vi "GetEvents_Motor Controller.vi"(8 "error in (no error)":errorcluster, 11 "TopLevel in":refnum<class "Motor Controller.lvclass">) -> (0 "error out":errorcluster, 2 "UserEvents":T1, 3 "TopLevel out":refnum<class "Motor Controller.lvclass">)   [LabVIEW 2022 SP3, in "Motor Controller.lvclass"]
uses:
  Motor Controller.lvclass
  Typedefs/UserEvents.ctl
  Typedefs/API Event Data.ctl
  Typedefs/API Task State.ctl
  Typedefs/Status.ctl
  TopLevel/Typedefs/Motor Controller Config Data.ctl
  Typedefs/Stage Move Data.ctl
  Typedefs/Batch Index Speed Data.ctl
  Typedefs/Move Status.ctl
  Motor Controller.lvclass/Motor Controller.ctl
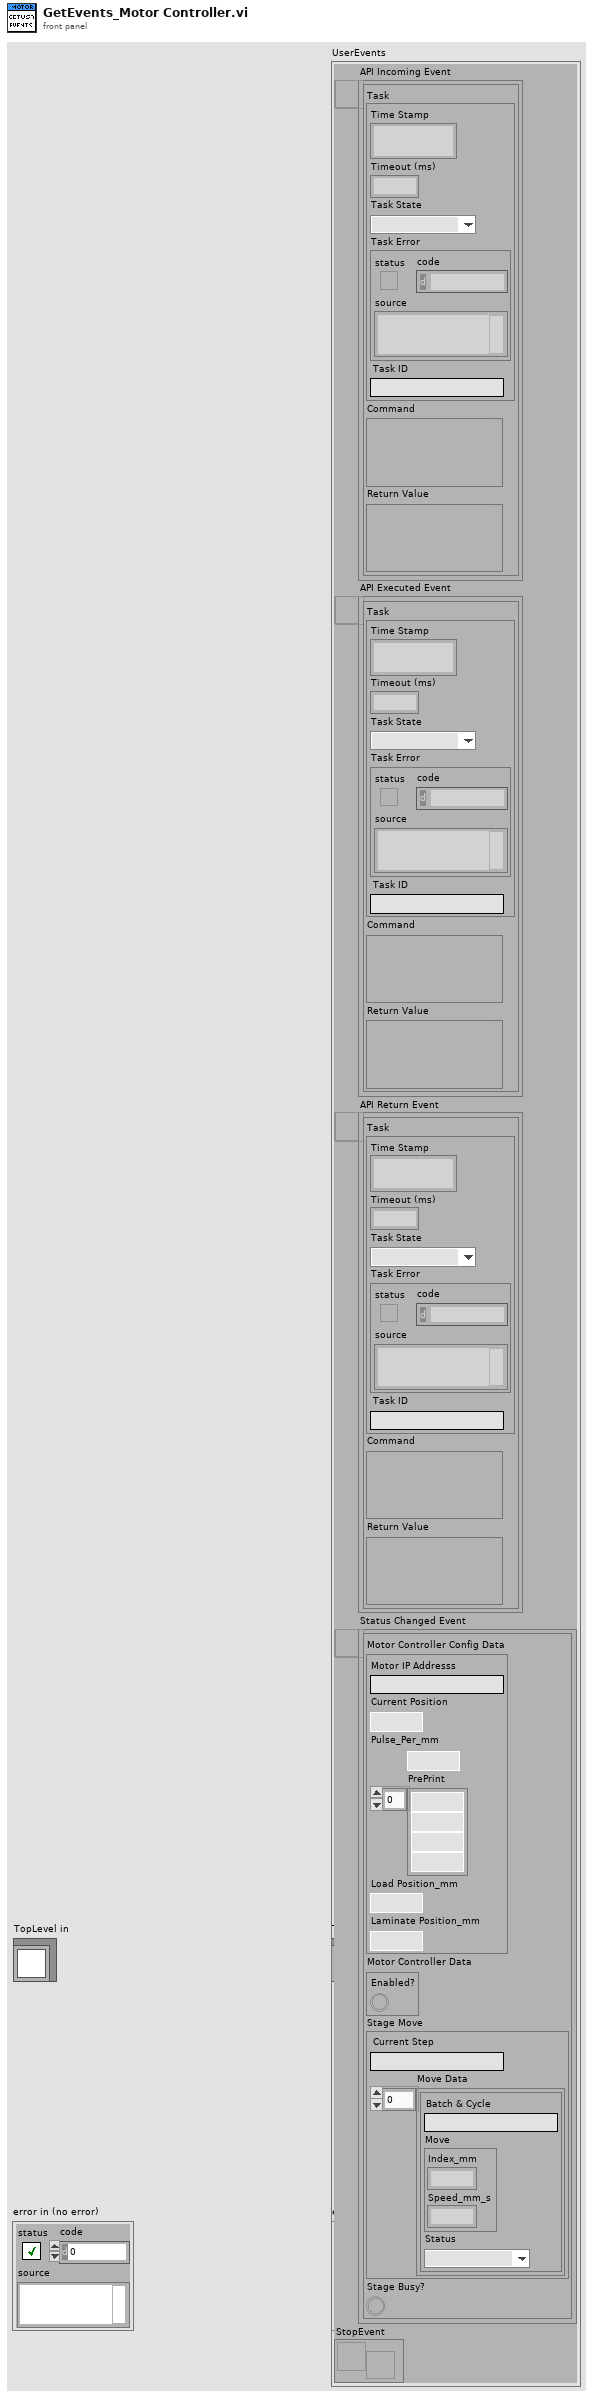
[diagram p1: front panel]
types:
  T1 = typedef "Motor Controller.lvclass/UserEvents.ctl" = cluster{"API Incoming Event":refnum<user-event>, "API Executed Event":refnum<user-event>, "API Return Event":refnum<user-event>, "Status Changed Event":refnum<user-event>, "StopEvent":refnum<user-event>}
  T2 = typedef "Motor Controller.lvclass/Private Data.ctl" = cluster{"UserEvents":T1, "All Dependencies":cluster{"Class References":refnum<class>[], "Class Names":string[]}, "Status":T3}
  T3 = typedef "Motor Controller.lvclass/Status.ctl" = cluster{"Motor Controller Config Data":T4, "Motor Controller Data":cluster{"Enabled?":bool}, "Stage Move":T5, "Stage Busy?":bool}
  T4 = typedef "Motor Controller.lvclass/Motor Controller Config Data.ctl" = cluster{"Motor IP Addresss":string, "Current Position":i32, "Pulse_Per_mm":i32, "PrePrint":dbl[], "Load Position_mm":i32, "Laminate Position_mm":i32}
  T5 = typedef "Motor Controller.lvclass/Stage Move Data.ctl" = cluster{"Current Step":string, "Move Data":T6[]}
  T6 = typedef "Motor Controller.lvclass/Batch Index Speed Data.ctl" = cluster{"Batch & Cycle":string, "Move":cluster{"Index_mm":i32, "Speed_mm_s":i32}, "Status":T7}
  T7 = typedef "Motor Controller.lvclass/Move Status.ctl" = enum16{"Pending", "In Progress", "Completed"}
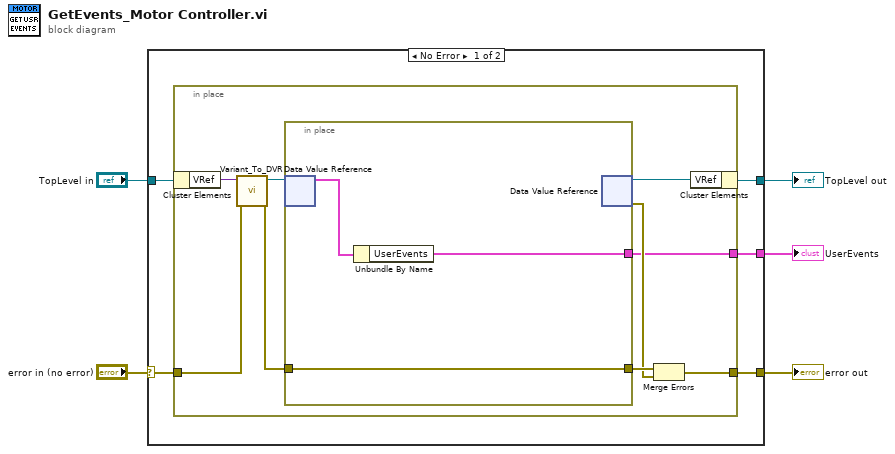
[diagram p0: block diagram]
diagram:
  n1 = case shown="No Error" "error in (no error)" {
    selector: "error in (no error)" -> [w7 w24]
    tunnel: [w9 w24] -> w4
    tunnel: [w10 w23] -> w2
    tunnel: "TopLevel in" -> [w8 w23]
    tunnel: [w6 _] -> w1
    frame No Error {
      n2 = in-place {
        in-place-border: w7 -> [w17]
        in-place-border: [w13] -> w9
        in-place-border: [w11] -> w6
        n3 = in-place-cluster #1(w8) -> ("VRef"=w19:variant)
        n4 = call "Variant_To_DVR.vi"("error in (no error)"=w17, "Variant"=w19) -> ("error out"=w16:errorcluster, "DVR"=w18:refnum<data-value>)  [unwired: 8 in]
        n5 = in-place {
          in-place-border: w16 -> [w21]
          in-place-border: [w21] -> w15
          in-place-border: [w20] -> w11
          n6 = in-place-dvr #2(w18) -> (w22:T2)  [unwired: 1 out]
          n7 = Unbundle By Name(w22) -> ("UserEvents"=w20:T1)
          n8 = in-place-dvr #2() -> (w12:refnum<data-value>, w14:errorcluster)  [unwired: 1 in]
        }
        n9 = Merge Errors(w15, w14) -> (w13:errorcluster)
        n10 = in-place-cluster #1("VRef"=w12) -> (w10:refnum<class "Motor Controller.lvclass">)
      }
    }
    frame Error {
    }
  }
  "error out" <- w4
  "TopLevel out" <- w2
  "UserEvents" <- w1
